vi "rebuild all.vi"() -> ()   [LabVIEW 2014]
uses:
  <vilib>/AppBuilder/AB_API_Simple/Build (path).vi
  <vilib>/AppBuilder/AB_API_Simple/NI_App_Builder_API.lvlib
panel:
  out "error":errorcluster
  in  "release (T) /debug (F)":bool
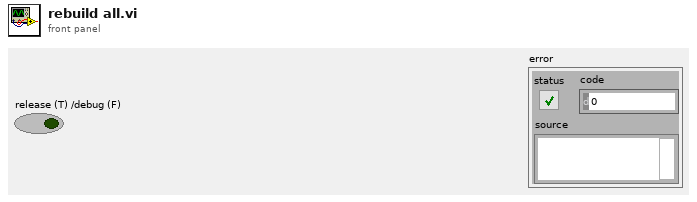
[diagram p1: front panel]
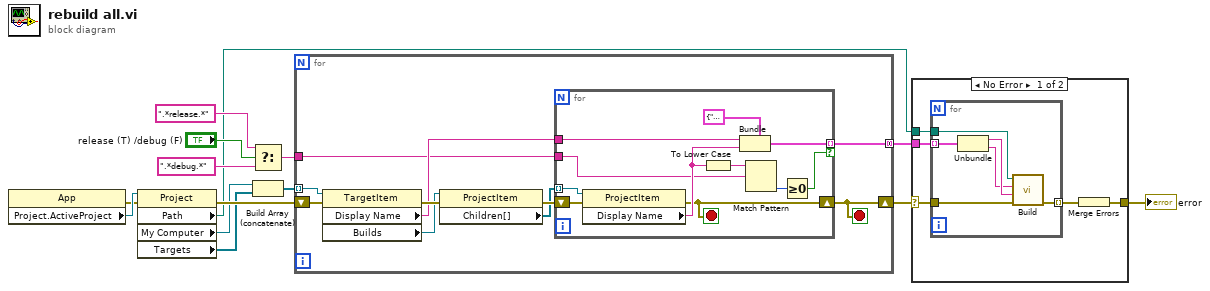
[diagram p0: block diagram]
diagram:
  n1 = property class="App"() -> (error out=w13:errorcluster, "Project.ActiveProject"=w14:refnum<vi>)  [unwired: 2 in, 1 out]
  n2 = property class="Project"(reference=w14, error in=w13) -> (error out=w12:errorcluster, "Path"=w3:path, "My Computer"=w11:refnum<vi>, "Targets"=w5:refnum<vi>[])  [unwired: 1 out]
  n3 = Select(t=".*release.*" ("regular expression"), s="release (T) /debug (F)", f=".*debug.*" ("regular expression")) -> (s? t:f=w7:string)
  n4 = Build Array (concatenate)(w11, w5) -> (w6:refnum<vi>[])
  n5 = for {
    tunnel: w7 -> [w21]
    tunnel: w6 -> [w20] mode=indexing
    shift-right: [w15] -> w2
    shift-left: w12 -> [w24]
    tunnel: [w19] -> w4 mode=concatenating
    stop <- w15 stop-if-true
    n6 = property class="TargetItem"(reference=w20, error in=w24) -> (error out=w23:errorcluster, "Display Name"=w22:string, "Builds"=w17:refnum<vi>)  [unwired: 1 out]
    n7 = property class="ProjectItem"(reference=w17, error in=w23) -> (error out=w18:errorcluster, "Children[]"=w16:refnum<vi>[])  [unwired: 1 out]
    n8 = for {
      shift-right: [w25] -> w15
      shift-left: w18 -> [w35]
      tunnel: w22 -> [w34]
      tunnel: [w32] -> w19 mode=indexing if=w30
      tunnel: w21 -> [w28]
      tunnel: w16 -> [w26] mode=indexing
      stop <- w25 stop-if-true
      n9 = property class="ProjectItem"(reference=w26, error in=w35) -> (error out=w25:errorcluster, "Display Name"=w33:string)  [unwired: 1 out]
      n10 = To Lower Case(string=w33) -> (all lower case string=w29:string)
      n11 = Bundle(cluster=cluster{"targ":string, "spec":string} {"targ"="", "spec"=""}, "targ"=w34, "spec"=w33) -> (w32:cluster{"targ":string, "spec":string})
      n12 = Match Pattern(string=w29, regular expression=w28) -> (offset past match=w31:i32)  [unwired: 1 in, 3 out]
      n13 = Greater Or Equal To 0?(x=w31) -> (x >= 0?=w30:bool)
    }
  }
  n14 = case shown="No Error" w2 {
    selector: w2 -> [w38 w47]
    tunnel: w4 -> [w40 _]
    tunnel: w3 -> [w39 _]
    tunnel: [w36 w47] -> w1
    frame No Error {
      n15 = for {
        tunnel: w40 -> [w43] mode=indexing
        tunnel: w39 -> [w46]
        tunnel: w38 -> [w45]
        tunnel: [w44] -> w37 mode=indexing
        n16 = Unbundle(w43) -> ("targ"=w42:string, "spec"=w41:string)
        n17 = call-poly <vilib>:"Build.vi"("error in (no error)"=w45, "Name of target (My Computer)"=w42, "Name of build specification (if empty: build all)"=w41, "Path to project"=w46) -> ("error out"=w44:errorcluster)  [unwired: 6 in, 1 out]
      }
      n18 = Merge Errors(w37) -> (w36:errorcluster)
    }
    frame Error {
    }
  }
  "error" <- w1
